vi "Default or Users Font, Leading and Alignment.vi"(0 "PDF Report":refnum<class "PDF Report Class.lvclass">, 5 "Font":T6={"Name"="", "Size"=-1.0, "Color"=0, "Style"={"Bold"=FALSE, "Italic"=FALSE, "Underline"=FALSE, "Strikeout"=FALSE}, "Type"={"Type&direction"=enum."Select", "Embedded"=FALSE, "Encoding"=""}}, 9 "Paragraphe cluster":T2, 11 "error in (no error)":errorcluster) -> (3 "Type and run direction":T1, 4 "PDF Report duplicate":refnum<class "PDF Report Class.lvclass">, 6 "Leading":T5=18.0, 8 "Font Ref":refnum<k24>, 10 "Close Font Ref":bool=TRUE, 14 "Aligment":string="JUSTIFY", 15 "error out":errorcluster)   [LabVIEW 2019, in "Exaprom PDF.lvlib"]
doc: "Version 2.0\nDeveloped by Jean-Marc Simard\nCopyright © 2012, Exaprom Inc.\nAll rights reserved.\nLicense: BSD\n\nWith iTextSharp 4.1.6 (http://itextsharp.sourceforge.net)\nunder Mozilla Public License Version 1.1\n(http://www.mozilla.org/MPL/MPL-1.1.html)"
uses:
  Exaprom PDF.lvlib
  LV Class/PDF Report Class/PDF Report Class.lvclass
  Controls/Font Controls/Font complete cluster.ctl
  Controls/Font Controls/Font size.ctl
  Controls/Font Controls/Font color.ctl
  Controls/Font Controls/Type and encoding.ctl
  Controls/Text Controls/Unicode/Type and run direction.ctl
  C:/work/niobrara_lv/labview pdf writer fixing/DLL/itextsharp.dll
  DLL/itextsharp.dll
  Controls/Initialization Controls/Defaut Paragraphe and Line Spacing.ctl
  Controls/Text Controls/Texte alignement.ctl
  Controls/Text Controls/Line spacing.ctl
  LV Class/Fonts Class/Font Class.lvclass
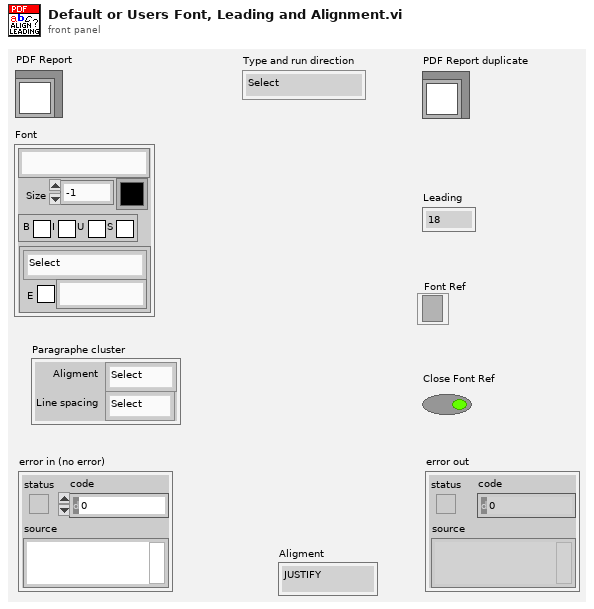
[diagram p1: front panel]
types:
  T1 = typedef "Exaprom PDF.lvlib/Type and run direction.ctl" = enum16{"Select", "ASCII", "UTF-16", "UTF-16 (default)", "UTF-16 (LTR)", "UTF-16 (RTL)"}
  T2 = typedef "Exaprom PDF.lvlib/Defaut Paragraphe and Line Spacing.ctl" = cluster{" Aligment":T3, "Line spacing":T4}
  T3 = typedef "Exaprom PDF.lvlib/Texte alignement.ctl" = enum16{"Select", "CENTER", "JUSTIFY", "LEFT", "RIGHT"}
  T4 = typedef "Exaprom PDF.lvlib/Line spacing.ctl" = enum16{"Select", "1.0", "1.5", "2.0"}
  T5 = typedef "Exaprom PDF.lvlib/Font size.ctl" = sgl
  T6 = typedef "Exaprom PDF.lvlib/Font complete cluster.ctl" = cluster{"Name":string, "Size":T5, "Color":T7, "Style":cluster{"Bold":bool, "Italic":bool, "Underline":bool, "Strikeout":bool}, "Type":T8}
  T7 = typedef "Exaprom PDF.lvlib/Font color.ctl" = u32
  T8 = typedef "Exaprom PDF.lvlib/Type and encoding.ctl" = cluster{"Type&direction":T1, "Embedded":bool, "Encoding":string}
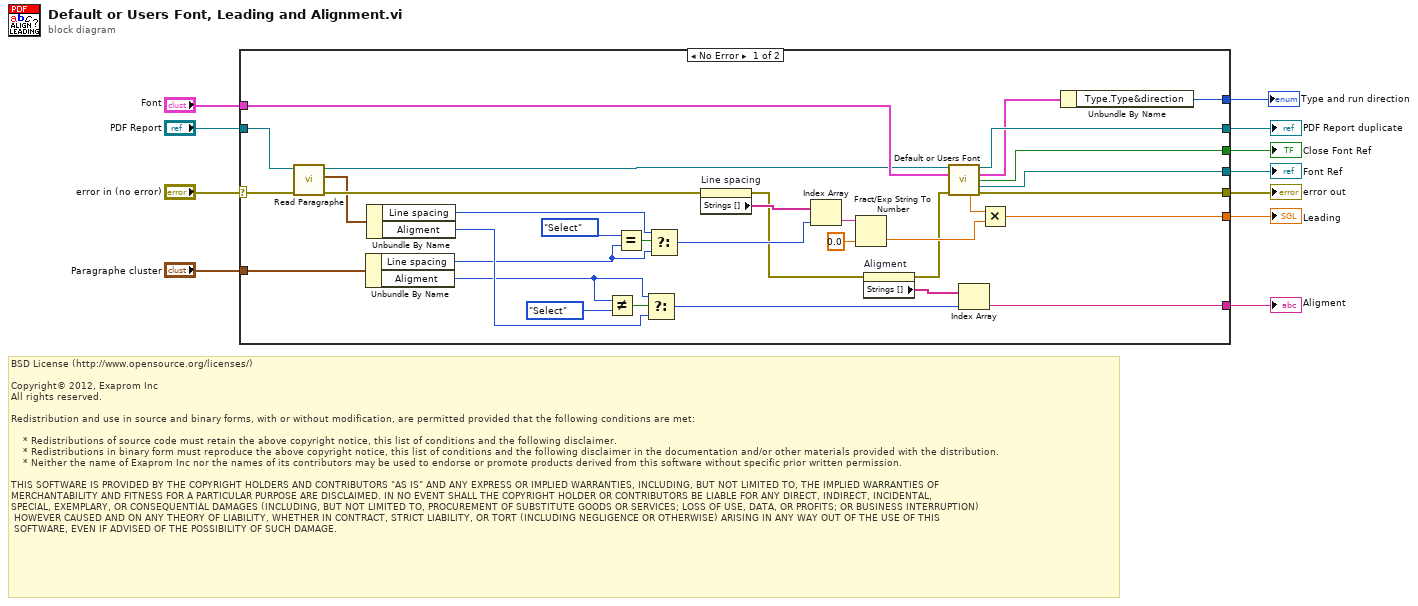
[diagram p0: block diagram]
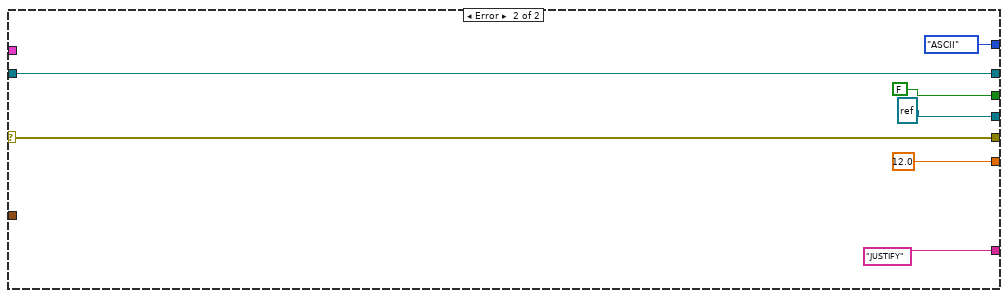
[diagram p2: hidden frame]
diagram:
  # "BSD License (http://www.opensource.org/licenses/)\n\nCopyright© 2012, Exaprom Inc\nAll rights reserved.\n\nRedistribution and use in source and binary forms, with or without modification, are permitted provided that the following conditions are met:\n\n    * Redistributions of source code must retain the above copyright notice, this list of conditions and the following disclaimer.\n    * Redistributions in binary form must reproduce the above copyright notice, this list of conditions and the following disclaimer in the documentation and/or other materials provided with the distribution.\n    * Neither the name of Exaprom Inc nor the names of its contributors may be used to endorse or promote products derived from this software without specific prior written permission.\n\nTHIS SOFTWARE IS PROVIDED BY THE COPYRIGHT HOLDERS AND CONTRIBUTORS \"AS IS\" AND ANY EXPRESS OR IMPLIED WARRANTIES, INCLUDING, BUT NOT LIMITED TO, THE IMPLIED WARRANTIES OF \nMERCHANTABILITY AND FITNESS FOR A PARTICULAR PURPOSE ARE DISCLAIMED. IN NO EVENT SHALL THE COPYRIGHT HOLDER OR CONTRIBUTORS BE LIABLE FOR ANY DIRECT, INDIRECT, INCIDENTAL,\nSPECIAL, EXEMPLARY, OR CONSEQUENTIAL DAMAGES (INCLUDING, BUT NOT LIMITED TO, PROCUREMENT OF SUBSTITUTE GOODS OR SERVICES; LOSS OF USE, DATA, OR PROFITS; OR BUSINESS INTERRUPTION)\n HOWEVER CAUSED AND ON ANY THEORY OF LIABILITY, WHETHER IN CONTRACT, STRICT LIABILITY, OR TORT (INCLUDING NEGLIGENCE OR OTHERWISE) ARISING IN ANY WAY OUT OF THE USE OF THIS\n SOFTWARE, EVEN IF ADVISED OF THE POSSIBILITY OF SUCH DAMAGE."
  n1 = case shown="No Error" "error in (no error)" {
    selector: "error in (no error)" -> [w18 w50]
    tunnel: [w44 "JUSTIFY"] -> w11
    tunnel: "Paragraphe cluster" -> [w43 _]
    tunnel: [w26 T5 12.0 ("Font Size")] -> w9
    tunnel: "PDF Report" -> [w15 w51]
    tunnel: [w25 w51] -> w7
    tunnel: "Font" -> [w24 _]
    tunnel: [w23 FALSE ("Close Font Ref")] -> w5
    tunnel: [w22 refnum<k24> refnum ("Font Ref")] -> w4
    tunnel: [w19 w50] -> w3
    tunnel: [w12 Type_and_run_direction."ASCII" ("Type&direction")] -> w1
    frame No Error {
      n2 = call-dynamic "Read Paragraphe.vi"("error in (no error)"=w18, "PDF Report Class in"=w15) -> ("error out"=w17:errorcluster, "Paragraphe cluster"=w16:T2, "PDF Report Class out"=w14:refnum<class "PDF Report Class.lvclass">)  [unwired: 7 in]
      n3 = Unbundle By Name(w43) -> ("Line spacing"=w33:T4, "Aligment"=w32:T3)
      n4 = Unbundle By Name(w16) -> ("Line spacing"=w35:T4, "Aligment"=w34:T3)
      n5 = Not Equal?(x=w32, y=Texte_alignement."Select" ("Aligment 2")) -> (x != y?=w37:bool)
      n6 = Equal?(x=Line_spacing."Select", y=w33) -> (x = y?=w39:bool)
      n7 = Select(t=w32, s=w37, f=w34) -> (s? t:f=w36:T3)
      n8 = Select(t=w35, s=w39, f=w33) -> (s? t:f=w38:T4)
      n9 = property on="Line spacing" class="Enum (strict)"(error in=w17) -> (error out=w29:errorcluster, "Strings []"=w30:string[])  [unwired: 1 in, 1 out]
      n10 = Index Array(array=w30, index=w38) -> (element=w41:string)
      n11 = Fract/Exp String To Number(string=w41, default (0 dbl)=sgl 0.0 ("default (0 DBL)")) -> (number=w27:sgl)  [unwired: 3 out]
      n12 = property on="Aligment" class="Enum (strict)"(error in=w29) -> (error out=w20:errorcluster, "Strings []"=w28:string[])  [unwired: 1 in, 1 out]
      n13 = call "Default or Users Font.vi"("PDF Report"=w14, "Font"=w24, "error in (no error)"=w20) -> ("PDF Report duplicate"=w25:refnum<class "PDF Report Class.lvclass">, "Font OUT"=w13:T6, "Close Font Ref"=w23:bool, "Font Ref"=w22:refnum<k24>, "Font Size"=w21:T5, "error out"=w19:errorcluster)  [unwired: 7 in]
      n14 = Index Array(array=w28, index=w36) -> (element=w44:string)
      n15 = Multiply(x=w21, y=w27) -> (x*y=w26:T5)
      n16 = Unbundle By Name(w13) -> ("Type.Type&direction"=w12:T1)
    }
    frame Error {
    }
  }
  "PDF Report duplicate" <- w7
  "error out" <- w3
  "Font Ref" <- w4
  "Leading" <- w9
  "Aligment" <- w11
  "Close Font Ref" <- w5
  "Type and run direction" <- w1
